vi "Komponentenausgabe_MG_HovaCAL.vi"(8 "error in (no error)":errorcluster caption="Fehler (Eingang, kein Fehler)") -> (0 "error out":errorcluster caption="Fehler (Ausgang)", 1 "Gasnummer out":u8, 2 "GesamtKonzentration":sgl, 3 "Gaskomponente":T2, 4 "Komponenten Name":T3, 5 "höchste Konzentration Teilkomponente ppm":dbl, 6 "Komponentenauswahl":T1 {"Konzentration" format="%#.6f"}, 7 "Component Index GD sorted":i32[](array[numeric]), 11 "GesamtKonzentration ppm":dbl)   [LabVIEW 2020, in "Linearisierung v2.lvlib"]
uses:
  Linearisierung v2.lvlib
  Visualisierungs Elemente/Auswahlfeld.ctl
  Visualisierungs Elemente/String - Ausgabefeld.ctl
  KomponentenArray.ctl
  Aktion Lin Daten aufarbeiten.ctl
  Gasteiler/Aktion FGV Gasteilerliste laden.ctl
  5aeeab1d-1b81-47b2-b563-9525e56eaefe.vi
  <vilib>/Array/Sort 2D Array - Pop Stack.vi
  <vilib>/Array/Sort 2D Array - Push Stack.vi
  5aeeab1d-1b81-47b2-b563-9525e56eaefe.vi/269d4b3b-47f5-49e3-8884-44851e4dd9d5.vi
  5aeeab1d-1b81-47b2-b563-9525e56eaefe.vi/6d99389c-673d-4efb-bf33-19b32bcf4cf8.vi
  Gasteiler/Gasteiler.lvlib
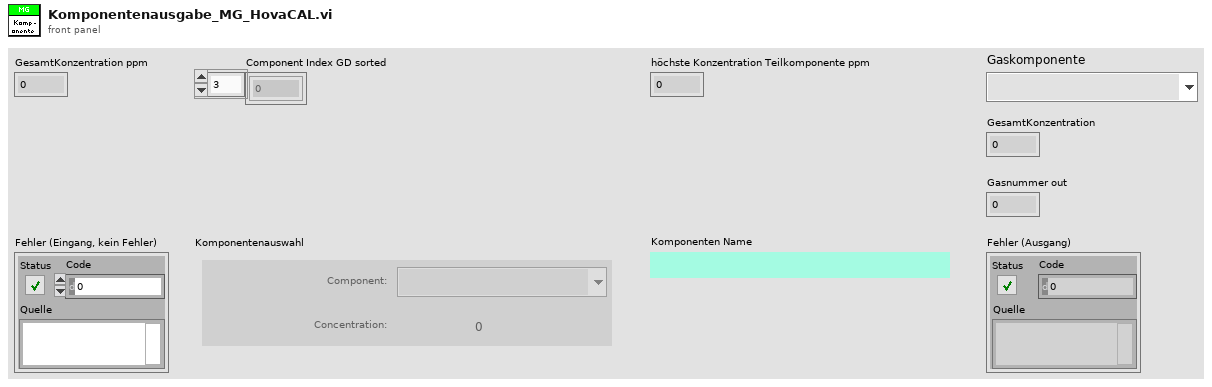
[diagram p1: front panel]
types:
  T1 = typedef "Linearisierung v2.lvlib/KomponentenArray.ctl" = cluster{"Komponente:":T2, "Konzentration":dbl}[]
  T2 = typedef "Auswahlfeld.ctl" = u16
  T3 = typedef "String - Ausgabefeld.ctl" = string
  T4 = typedef "Linearisierung v2.lvlib/Aktion Lin Daten aufarbeiten.ctl" = enum16{"lesen", "Protkolldaten", "speichern", "laden", "EPA auswerten", "Tabelle schreiben", "Lin auswerten", "Tab init", "Stufentabelle", "EPA aktiviert", "Nachbehandlung laden", "Tabelle löschen", "Istwerte löschen", "Zeile löschen", "Zeile einfügen", "LIN aktiviert", "LIN/EPA aktiv laden", "EGAK Tab", "LIN übernehmen", "Tab init ohne Stufen"}
  T5 = typedef "Linearisierung v2.lvlib/Lin-Polynom Daten.ctl" = cluster{"Messgerät":string, "Kalibrator (Gasteiler)":string, "Bearbeiter/in":string, "Komponente":string, "Zeitstempel":timestamp, "F_max gefordert (%)":sgl, "F_max in %":sgl, "F_max in ppm":sgl, "Vorschlag Ordnung":i32, "Polynom OK":bool, "Polynomkoeff.":dbl[], "Prüfgas Konzentration":dbl, "Pfad EPA":string, "Pfad_LIN":string, "Gasnummer:":u8, "Komponentenauswahl":T1, "Verdünnungsgas":T6, "Zeitdauer Stufe":T7, "Anzahl Stufen":T7, "F_max in % EPA":sgl, "F_max in ppm EPA":sgl, "F_max in % LIN":sgl, "F_max in ppm LIN":sgl, "Punkte umkehren":bool, "EPA Optionsfeld":T8, "Autolin Hovacal":T9, "Spanfactors":sgl[], "Kalibrierauswahl":T10, "Conditions:":T11, "Gasflaschen Nr.:":string, "Bottle Accuracy":dbl, "Konfig Gasflasche":T12, "Gasflasche":T13, "HovaCAL Flow AutoLin":T14, "MFC Output":T15, "Gas Ablaufdatum":timestamp, "Lin Modus":T16, "zusätzliche Zeitdauer Erster Punkt":sgl, "Offsets":sgl[]}
  T6 = typedef "Linearisierung v2.lvlib/Gasteiler.lvlib/Prüfgas in.ctl" = u16
  T7 = typedef "Zahlen-Eingabefeld.ctl" = sgl
  T8 = typedef "Linearisierung v2.lvlib/EPA Optionsfeld.ctl" = enum32{"Istwert", "Rohwert", "Linearisierter Wert"}
  T9 = typedef "Linearisierung v2.lvlib/Gasteiler.lvlib/HovaCal.lvlib/AutoLin Hovacal.ctl" = enum32{"Keine Auswahl", "Optionsauswahl 1", "Optionsauswahl 2"}
  T10 = typedef "Linearisierung v2.lvlib/Kalibrieroption.ctl" = u16
  T11 = typedef "Linearisierung v2.lvlib/Linearity verification 1065-307.lvlib/Condition.ctl" = u16
  T12 = typedef "System Einstellungen V2.lvlib/Konfig Gasflasche.ctl" = bool
  T13 = typedef "System Einstellungen V2.lvlib/Gasflasche Auswahl.ctl" = u16
  T14 = typedef "Linearisierung v2.lvlib/Gasteiler.lvlib/HovaCAL_Interface.lvlib/Controls.lvlib/Flow Einstellung.ctl" = cluster{"HovaCAL Flow Input Cluster":dbl}
  T15 = typedef "Linearisierung v2.lvlib/Gasteiler.lvlib/HovaCAL_Interface.lvlib/Controls.lvlib/Pump state.ctl" = cluster{"Run":bool}
  T16 = typedef "CalGas Aufschaltung.lvlib/Lin Modus.ctl" = u16
  T17 = typedef "Linearisierung v2.lvlib/Gasteiler.lvlib/Aktion FGV Gasteilerliste laden.ctl" = enum16{"lesen", "laden", "speichern", "Liste erstellen", "Formel ändern", "Gas vereinzeln"}
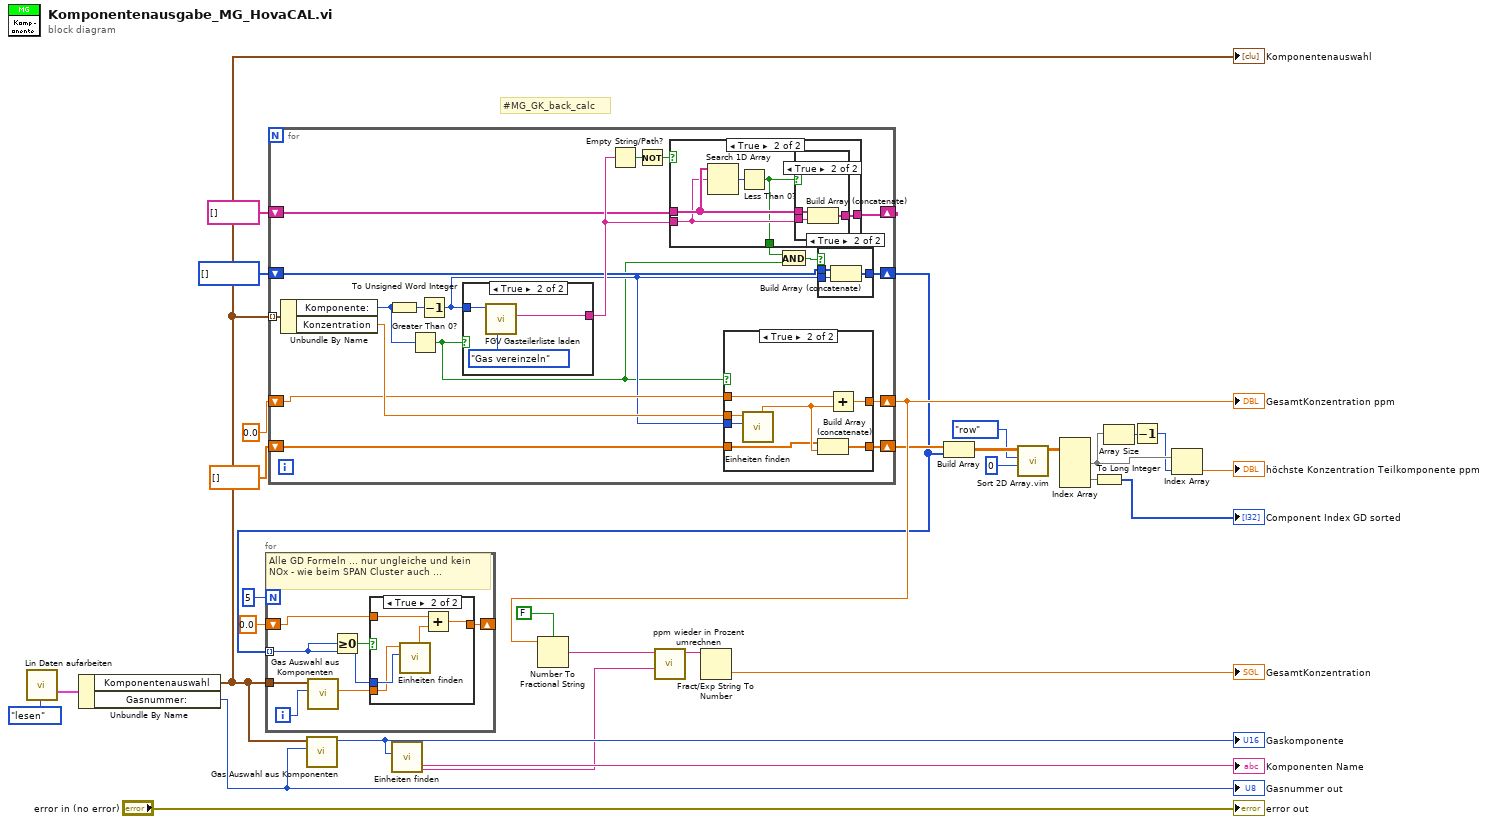
[diagram p0: block diagram]
diagram:
  w21 = T2[] [] items=[""]
  # "#MG_GK_back_calc"
  n1 = call "Lin Daten aufarbeiten.vi"("Aktionen"=Aktion_Lin_Daten_aufarbeiten."lesen") -> ("Lin-Polynom"=w30:T5)  [unwired: 16 in, 10 out]
  n2 = Unbundle By Name(w30) -> ("Komponentenauswahl"=w23:T1, "Gasnummer:"=w26:u8)
  "Gasnummer out" <- w26
  "Komponentenauswahl" <- w23
  n3 = for {
    tunnel: w23 -> [w50] mode=indexing
    shift-right: [w45] -> _
    shift-left: string[] [] -> [w43]
    shift-right: [w40] -> w2
    shift-left: w21 -> [w39]
    shift-right: [w37] -> w18
    shift-left: 0.0 -> [w36]
    shift-right: [w33] -> w3
    shift-left: dbl[] [] -> [w32]
    n4 = Unbundle By Name(w50) -> ("Komponente:"=w48:T2, "Konzentration"=w38:dbl)
    n5 = To Unsigned Word Integer(number=w48) -> (unsigned 16bit integer=w49:T2)
    n6 = Greater Than 0?(x=w48) -> (x > 0?=w34:bool)
    n7 = Decrement(x=w49) -> (x-1=w35:T2)
    n8 = case shown="True" w34 {
      tunnel: w35 -> [_ w76]
      tunnel: [_ w75] -> w44
      frame False {
      }
      frame True {
        n9 = call "FGV Gasteilerliste laden.vi"("Aktion"=Aktion_FGV_Gasteilerliste_laden."Gas vereinzeln", "Gasindex"=w76) -> ("Formel"=w75:string)  [unwired: 7 in, 2 out]
      }
    }
    n10 = Empty String/Path?(string/path=w44) -> (empty?=w47:bool)
    n11 = Not(x=w47) -> (.not. x?=w46:bool)
    n12 = case shown="True" w46 {
      selector: w46 -> [w64 _]
      tunnel: [w65 w70] -> w45
      tunnel: w43 -> [w65 w69]
      tunnel: w44 -> [_ w68]
      tunnel: [w64 w66] -> w42
      frame False {
      }
      frame True {
        n13 = Search 1D Array(1D array=w69, element=w68) -> (index of element=w67:i32)  [unwired: 1 in]
        n14 = Less Than 0?(x=w67) -> (x < 0?=w66:bool)
        n15 = case shown="True" w66 {
          tunnel: [w71 w74] -> w70
          tunnel: w69 -> [w71 w73]
          tunnel: w68 -> [_ w72]
          frame False {
          }
          frame True {
            n16 = Build Array (concatenate)(w73, w72) -> (w74:string[])
          }
        }
      }
    }
    n17 = case shown="True" w34 {
      tunnel: w38 -> [_ w56]
      tunnel: [w52 w59] -> w37
      tunnel: w36 -> [w52 w58]
      tunnel: w35 -> [_ w57]
      tunnel: [w51 w54] -> w33
      tunnel: w32 -> [w51 w53]
      frame False {
      }
      frame True {
        n18 = call "Einheiten finden.vi"("Komponente"=w57, "Wert"=w56) -> ("Wert ppm"=w55:dbl)  [unwired: 5 in, 4 out]
        n19 = Build Array (concatenate)(w53, w55) -> (w54:dbl[])
        n20 = Add(x=w58, y=w55) -> (x+y=w59:dbl)
      }
    }
    n21 = And(x=w42, y=w34) -> (x .and. y?=w41:bool)
    n22 = case shown="True" w41 {
      tunnel: w35 -> [_ w63]
      tunnel: [w60 w62] -> w40
      tunnel: w39 -> [w60 w61]
      frame False {
      }
      frame True {
        n23 = Build Array (concatenate)(w61, w63) -> (w62:T2[])
      }
    }
  }
  "GesamtKonzentration ppm" <- w18
  n24 = for {
    N: 5 -> [_]
    tunnel: w23 -> [w84]
    shift-right: [w81] -> _
    shift-left: 0.0 -> [w80]
    tunnel: w2 -> [w78] mode=indexing
    i -> [w83]
    # "Alle GD Formeln ... nur ungleiche und kein NOx - wie beim SPAN Cluster auch ..."
    n25 = call "Gas Auswahl aus Komponenten.vi"("Gasnummer:"=w83, "Komponentenauswahl"=w84) -> ("Konzentration"=w82:dbl)  [unwired: 7 in, 2 out]
    n26 = Greater Or Equal To 0?(x=w78) -> (x >= 0?=w79:bool)
    n27 = case shown="True" w79 {
      tunnel: w78 -> [_ w90]
      tunnel: w82 -> [_ w89]
      tunnel: [w85 w87] -> w81
      tunnel: w80 -> [w85 w86]
      frame False {
      }
      frame True {
        n28 = call "Einheiten finden.vi"("Komponente"=w90, "Wert"=w89) -> ("Wert ppm"=w88:dbl)  [unwired: 5 in, 4 out]
        n29 = Add(x=w86, y=w88) -> (x+y=w87:dbl)
      }
    }
  }
  n30 = call "Gas Auswahl aus Komponenten.vi"("Gasnummer:"=w26, "Komponentenauswahl"=w23) -> ("Auswahl"=w25:T2)  [unwired: 7 in, 2 out]
  "Gaskomponente" <- w25
  n31 = call "Einheiten finden.vi"("Komponente"=w25) -> ("Einheit in String"=w19:string, "Komponenten Name"=→"Komponenten Name":T3)  [unwired: 6 in, 3 out]
  n32 = Number To Fractional String(use system decimal point (T)=FALSE ("Systemdezimalzeichen verwenden (T)"), number=w18) -> (F-format string=w16:string)  [unwired: 2 in]
  n33 = call "ppm wieder in Prozent umrechnen.vi"("Einheit"=w19, "Werteingang"=w16) -> ("Wertausgang"=w15:string)  [unwired: 9 in]
  n34 = Fract/Exp String To Number(string=w15) -> (number=→"GesamtKonzentration":dbl)  [unwired: 3 in, 1 out]
  n35 = Build Array(w3, w2) -> (w12:dbl[][])
  n36 = call "Sort 2D Array.vim"("index"=0, "dimension to index (column)"=enum16{"column", "row"}."row", "2D array"=w12) -> ("sorted 2D array"=w9:dbl[][])  [unwired: 7 in, 1 out]
  n37 = Index Array(array=w9) -> (element #1=w7:dbl[], element #2=w8:dbl[])  [unwired: 4 in]
  n38 = To Long Integer(number=w8) -> (32bit integer=→"Component Index GD sorted":i32[])
  n39 = Array Size(array=w7) -> (size(s)=w6:i32)
  n40 = Decrement(x=w6) -> (x-1=w5:i32)
  n41 = Index Array(array=w7, index=w5) -> (element=→"höchste Konzentration Teilkomponente ppm":dbl)
  "error out" <- "error in (no error)"
